vi "Remove Waveform.vi"(8 "error in":errorcluster, 10 "Waveforms UI Ctrl Ref":T2, 11 "Waveform Meas Config Ctrl Ref":T1) -> (0 "error out":errorcluster)   [LabVIEW 2025, in "Fgen Script Mode UI.lvlib"]
uses:
  Typedef/Waveforms UI Ctrl Ref.ctl
  Typedef/Waveform Meas Config Ctrl Ref.ctl
  Fgen Script Mode UI.lvlib
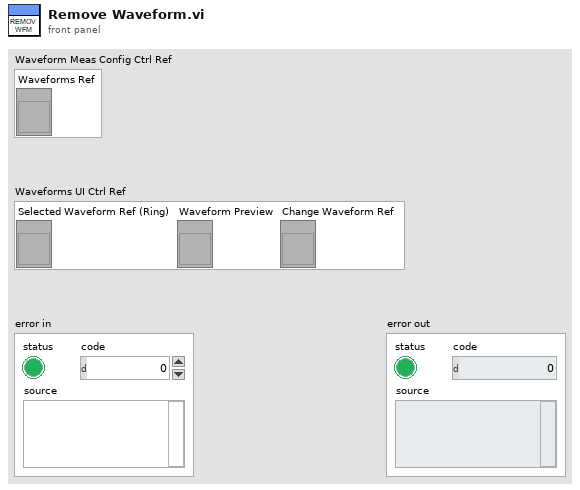
[diagram p1: front panel]
types:
  T1 = typedef "Fgen Script Mode UI.lvlib/Waveform Meas Config Ctrl Ref.ctl" = cluster{"Waveforms Ref":refnum<vi>}
  T2 = typedef "Fgen Script Mode UI.lvlib/Waveforms UI Ctrl Ref.ctl" = cluster{"Selected Waveform Ref (Ring)":refnum<vi>, "Waveform Preview":refnum<vi>, "Change Waveform Ref":refnum<vi>}
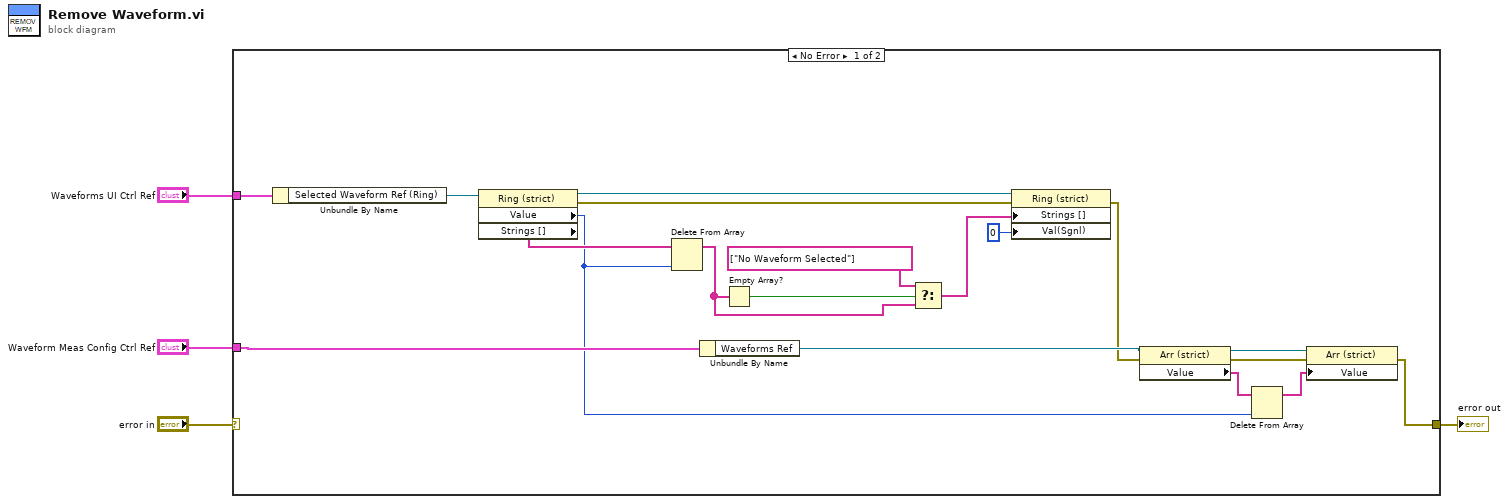
[diagram p0: block diagram]
diagram:
  n1 = case shown="No Error" "error in" {
    selector: "error in" -> [_ w24]
    tunnel: [w9 w24] -> w3
    tunnel: "Waveform Meas Config Ctrl Ref" -> [w10 _]
    tunnel: "Waveforms UI Ctrl Ref" -> [w23 _]
    frame No Error {
      n2 = Unbundle By Name(w23) -> ("Selected Waveform Ref (Ring)"=w22:refnum<vi>)
      n3 = property class="Ring (strict)"(reference=w22) -> (reference out=w18:refnum<vi>, error out=w17:errorcluster, "Value"=w5:u16, "Strings []"=w19:string[])  [unwired: 1 in]
      n4 = Delete From Array "Delete From Array"(array=w19, index=w5) -> (array with subset deleted=w16:string[])  [unwired: 1 in, 1 out]
      n5 = Unbundle By Name(w10) -> ("Waveforms Ref"=w21:refnum<vi>)
      n6 = Empty Array?(array=w16) -> (empty?=w12:bool)
      n7 = Select(t=string[] ["No Waveform Selected"] ("Strings []"), s=w12, f=w16) -> (s? t:f=w14:string[])
      n8 = property class="Ring (strict)"(reference=w18, error in=w17, "Strings []"=w14, "Val(Sgnl)"=u16 0 ("Value")) -> (error out=w11:errorcluster)  [unwired: 1 out]
      n9 = property class="Arr (strict)"(reference=w21, error in=w11) -> (reference out=w8:refnum<vi>, error out=w20:errorcluster, "Value"=w7:string[])
      n10 = Delete From Array(array=w7, index=w5) -> (array with subset deleted=w6:string[])  [unwired: 1 in, 1 out]
      n11 = property class="Arr (strict)"(reference=w8, error in=w20, "Value"=w6) -> (error out=w9:errorcluster)  [unwired: 1 out]
    }
    frame Error {
    }
  }
  "error out" <- w3
